vi "limit_deadband.vi"(5 "lower limit":dbl=-0.15, 7 "upper limit":dbl=0.15, 11 "Val":dbl) -> (3 "Val Out":dbl)   [LabVIEW 2015]
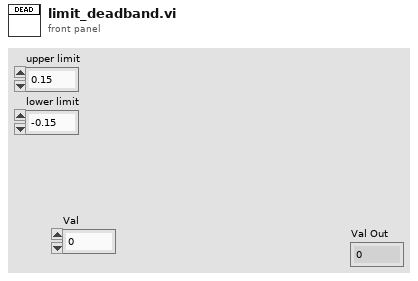
[diagram p1: front panel]
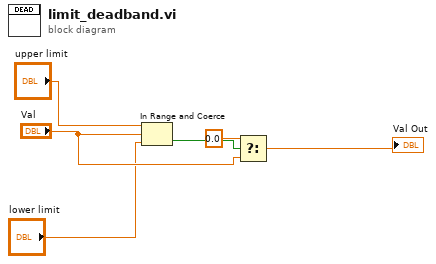
[diagram p0: block diagram]
diagram:
  n1 = In Range and Coerce(upper limit="upper limit", x="Val", lower limit="lower limit") -> (In Range?=w6:bool)  [unwired: 1 out]
  n2 = Select(t=0.0, s=w6, f="Val") -> (s? t:f=→"Val Out":dbl)
